vi "EKGTest.vi"() -> ()   [LabVIEW 2010]
uses:
  <instrlib>/niHWS/nihws.llb/niHWS Open File Permissions ID.ctl
  Fear Conditioning/GlobalFear.vi
  <instrlib>/niHWS/nihws.llb/niHWS Write Digital U32.vi
  <instrlib>/niHWS/nihws.llb/niHWS Write Analog DBL.vi
  <instrlib>/niHWS/nihws.llb/niHWS Write Analog WDT.vi
  <vilib>/measure/matone.llb/Extract Single Tone Information N Chan.vi
  <vilib>/measure/NI_MAPro.lvlib
panel:
  out "HR 3":dbl
  in  "Knob":dbl(knob) scale=7.0..15.0
  in  "stop":bool
  out "Filtered ECG Signal":waveform(dbl)[](graph)
  out "HR 2":dbl(graph)
  out "HR":dbl format="%#_4g"
  out "Detected HR":dynamicdata(graph)
  in  "HR % Change\nThreshold":dbl(slide)=25.0 scale=0.0..25.0
  out "Threshold":dbl
  out "Error Thr":dbl
  out "Skipped":bool
  in  "Rate Corrector":bool=TRUE
  in  "# average":dbl=20.0
  out "RAW ECG Signal":dynamicdata(graph)
  out "det Freq":dbl
  in  "Record":bool
  in  "Recording Path":path
  in  "Activity mouse":refnum<visa-resource-name>
  out "Activity monitor":dynamicdata(graph)
  in  "Mouse Axis":bool
  in  "DPI":dbl=350.0
  out "Cycles \ncompleted":dbl
  out "Shock":bool
  out "Audio":bool
  in  "Start":bool
  in  "stop 2":bool
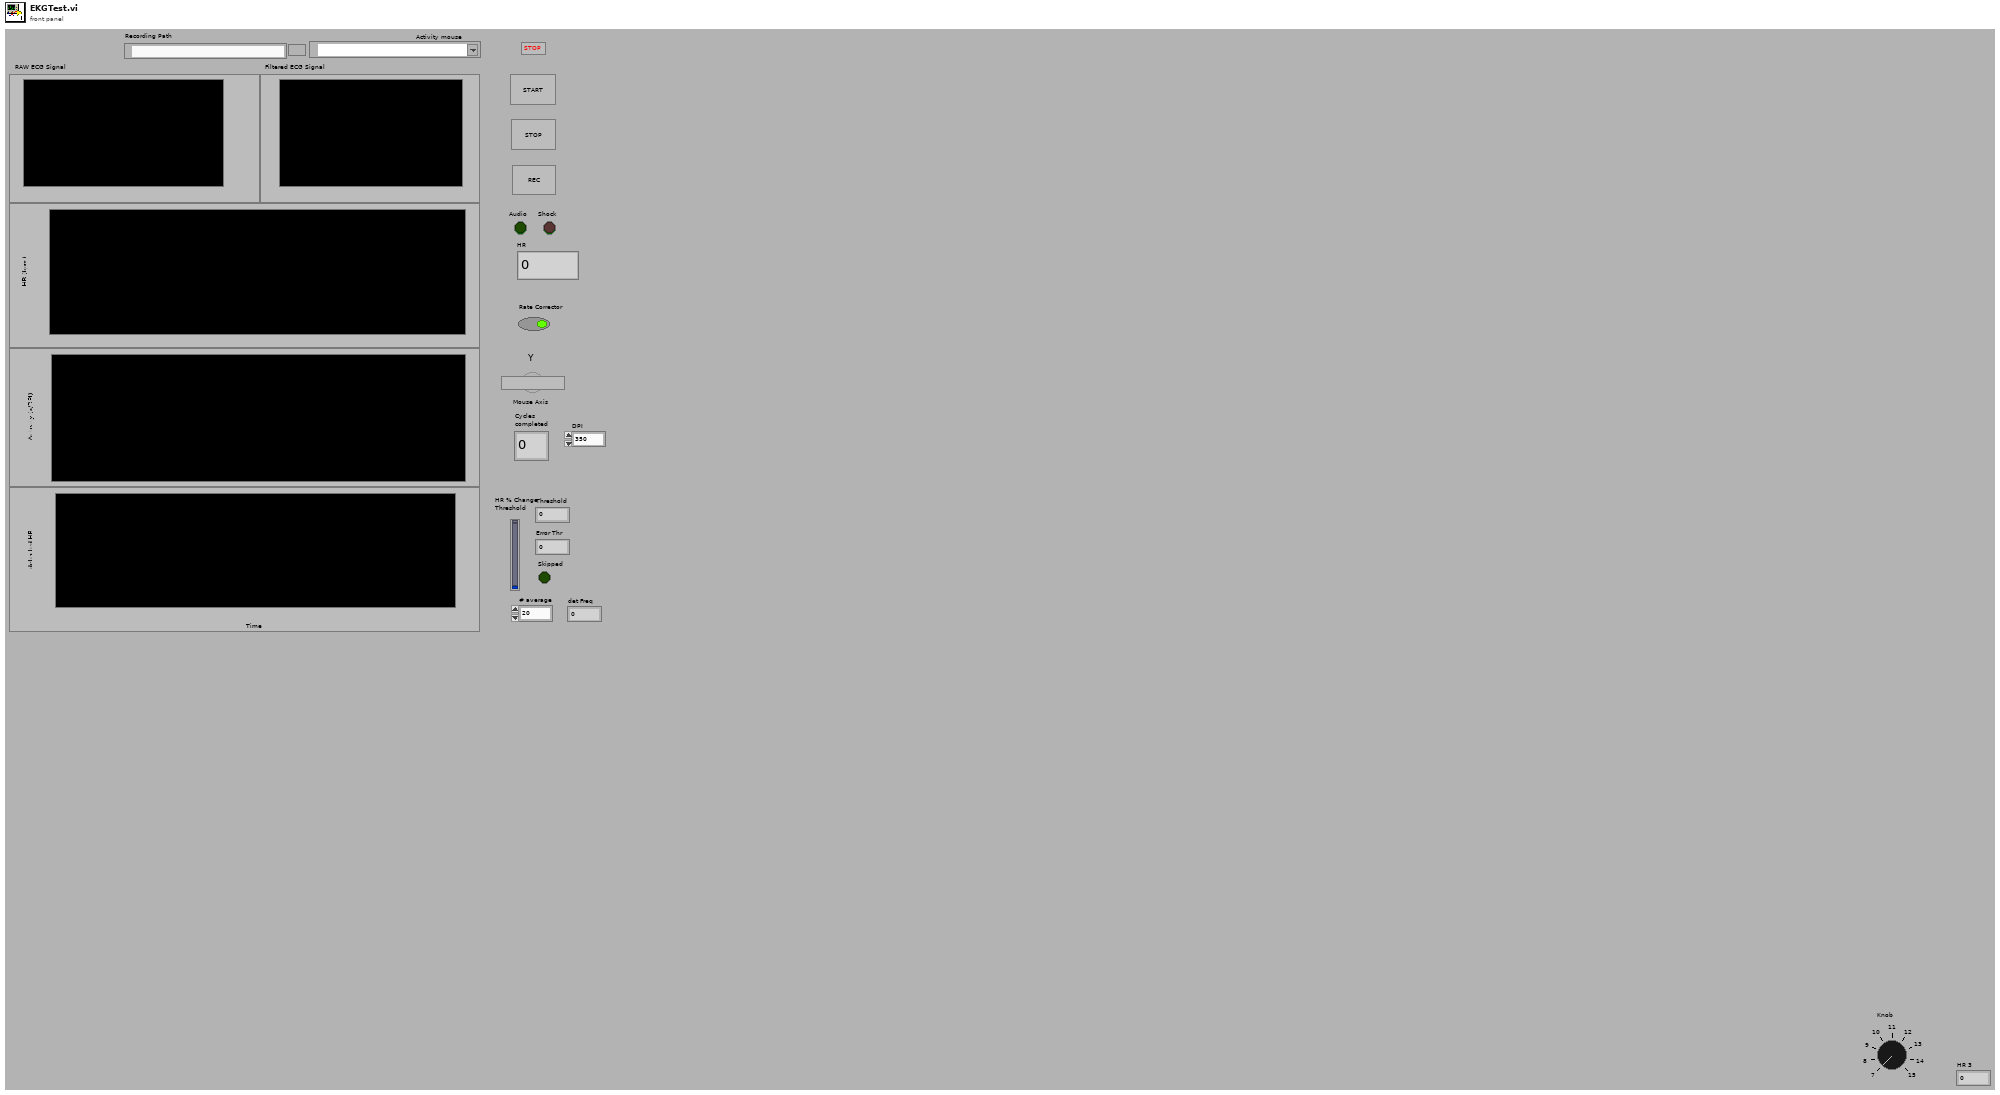
[diagram p1: front panel]
types:
  T1 = typedef "niHWS Open File Permissions ID.ctl" = enum32{"Read Only", "Read/Write Existing", "Read/Write/Create New", "Read/Write/Create New Always"}
  T2 = cluster{"approx freq. (optional)":dbl, "search (+/- % of Fsampl.)":dbl}
  T3 = cluster{"Array":dbl[], "Array 2":dbl[], "Array 3":dbl[], "Array 4":dbl[], "Array 5":dbl[], "Array 6":dbl[], "Array 7":dbl[], "Array 8":dbl[]}
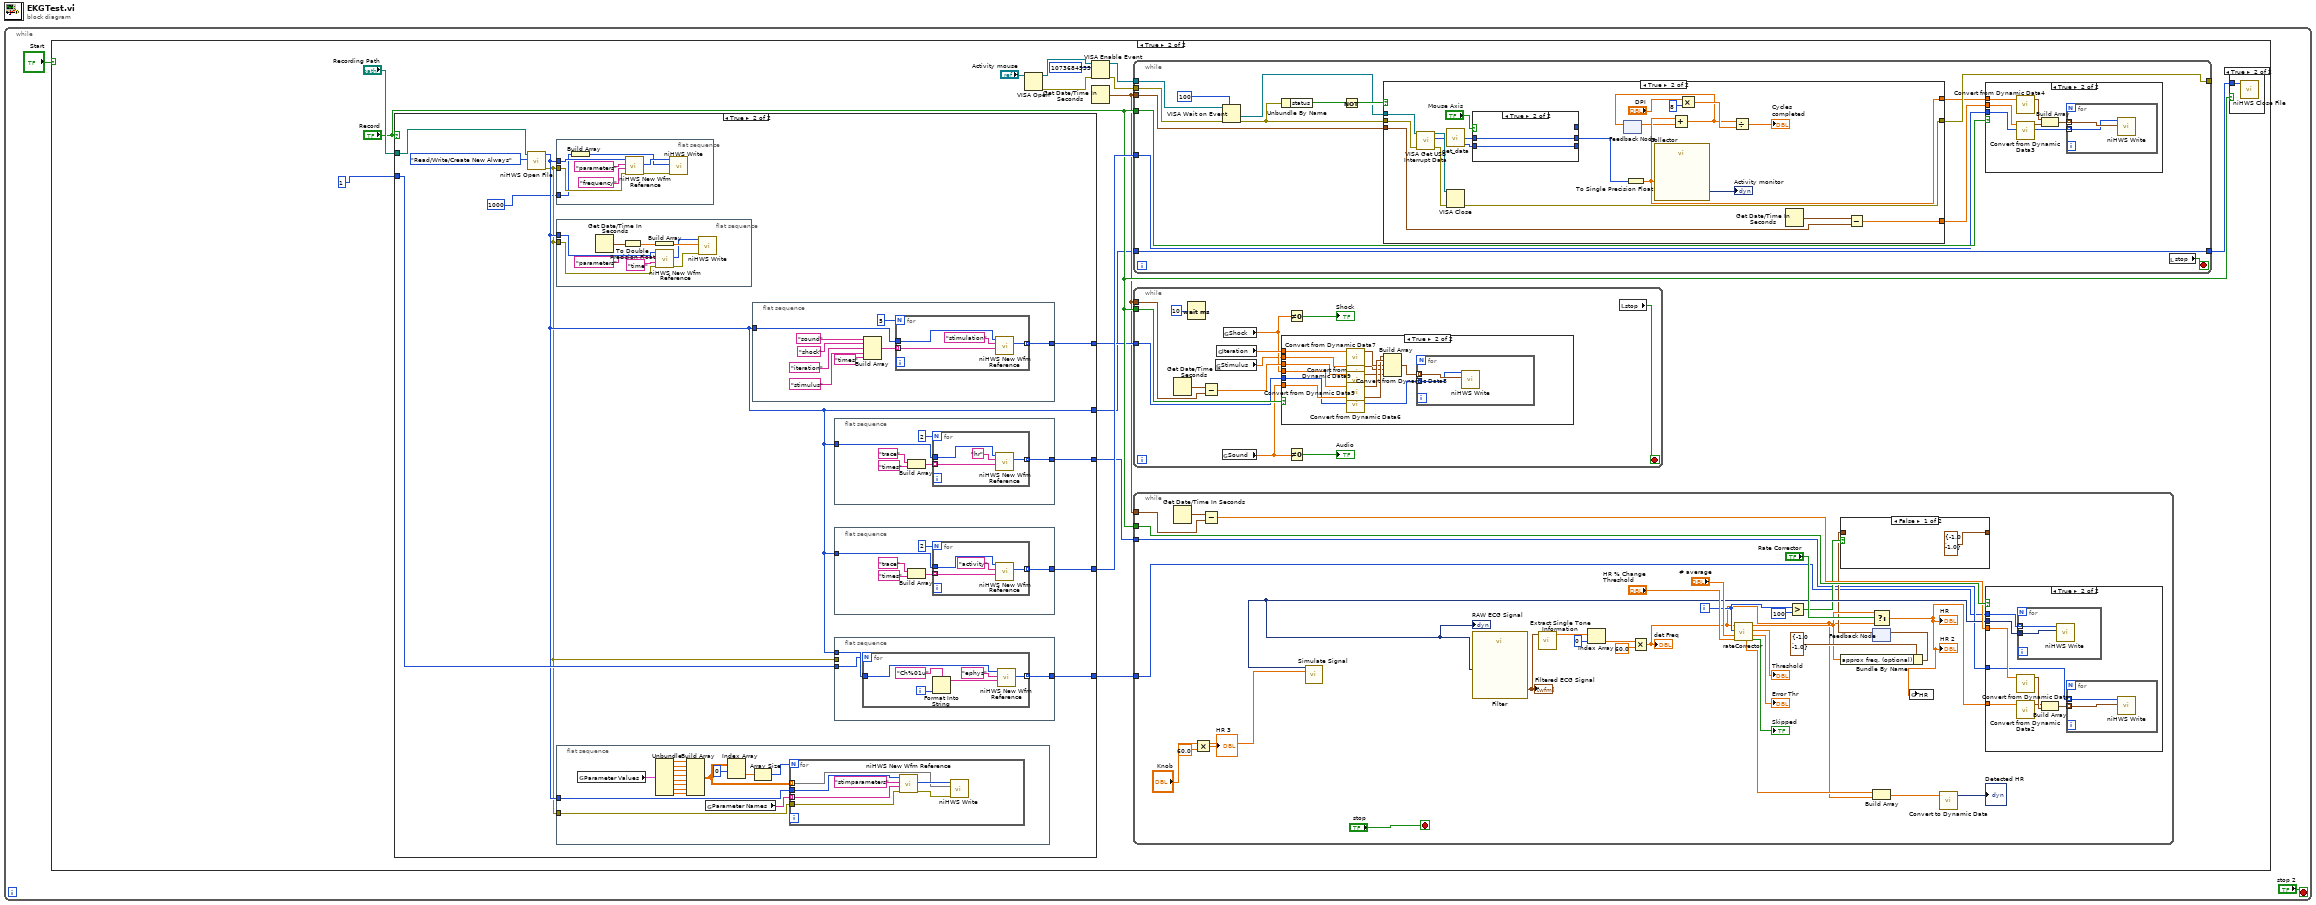
[diagram p0: block diagram]
diagram:
  n1 = while {
    stop <- "stop 2" stop-if-true
    n2 = case shown="True" "Start" {
      frame False {
      }
      frame True {
        n3 = case shown="True" "Record" {
          tunnel: 1 -> [_ w101]
          tunnel: "Recording Path" -> [_ w105]
          tunnel: [_ w103] -> w11
          tunnel: [_ w102] -> w9
          tunnel: [_ w99] -> w7
          tunnel: [_ w100] -> w5
          tunnel: [_ w97] -> w4
          frame False {
          }
          frame True {
            n4 = call <instrlib>:"niHWS Open File.vi"("permissions (0:read only)"=niHWS_Open_File_Permissions_ID."Read/Write/Create New Always", "file path"=w105) -> ("error out"=w98:errorcluster, "file handle"=w99:u32)  [unwired: 8 in]
            n5 = flat-sequence {
              tunnel: w98 -> [w160]
              tunnel: w99 -> [w159]
              tunnel: 1000 -> [w157]
              frame #0 {
                n6 = Build Array(w157) -> (w161:i32[])
                n7 = call <instrlib>:"niHWS New Wfm Reference.vi"("error in (no error)"=w160, "waveform name (empty)"="frequency" ("group name (empty)"), "group name (empty)"="parameters", "file handle in"=w159) -> ("error out"=w158:errorcluster, "waveform reference"=w164:u32)  [unwired: 5 in, 1 out]
                n8 = call-poly <instrlib>:"niHWS Write.vi"("error in (no error)"=w158, "data"=w161, "waveform reference in"=w164) -> ()  [unwired: 7 in, 2 out]
              }
            }
            n9 = flat-sequence {
              tunnel: w98 -> [w156]
              tunnel: w99 -> [w155]
              frame #0 {
                n10 = Get Date/Time In Seconds() -> (seconds since 1Jan1904=w154:timestamp)
                n11 = To Double Precision Float(number=w154) -> (double precision float=w153:dbl)
                n12 = Build Array(w153) -> (w152:dbl[])
                n13 = call <instrlib>:"niHWS New Wfm Reference.vi"("error in (no error)"=w156, "waveform name (empty)"="time" ("group name (empty)"), "group name (empty)"="parameters", "file handle in"=w155) -> ("error out"=w148:errorcluster, "waveform reference"=w149:u32)  [unwired: 5 in, 1 out]
                n14 = call-poly <instrlib>:"niHWS Write.vi"("error in (no error)"=w148, "data"=w152, "waveform reference in"=w149) -> ()  [unwired: 7 in, 2 out]
              }
            }
            n15 = flat-sequence {
              tunnel: w99 -> [w166]
              tunnel: w98 -> [w165]
              frame #0 {
                n16 = global read "GlobalFear.vi" "Parameter Values"() -> (w167:T3)
                n17 = Unbundle(w167) -> ("Array"=w168:dbl[], "Array 2"=w169:dbl[], "Array 3"=w170:dbl[], "Array 4"=w171:dbl[], "Array 5"=w172:dbl[], "Array 6"=w173:dbl[], "Array 7"=w174:dbl[], "Array 8"=w175:dbl[])
                n18 = Build Array(w168, w169, w170, w171, w172, w173, w174, w175) -> (w179:dbl[][])
                n19 = global read "GlobalFear.vi" "Parameter Names"() -> (w180:string[])
                n20 = Index Array(array=w179, index (row)=0) -> (element=w177:dbl[])  [unwired: 1 in]
                n21 = Array Size(array=w177) -> (size(s)=w176:i32)
                n22 = for {
                  N: w176 -> [_]
                  tunnel: w179 -> [w185] mode=indexing
                  tunnel: w180 -> [w184] mode=indexing
                  tunnel: w166 -> [w183]
                  tunnel: w165 -> [w182]
                  n23 = call <instrlib>:"niHWS New Wfm Reference.vi"("error in (no error)"=w182, "waveform name (empty)"=w184, "group name (empty)"="stimparameters", "file handle in"=w183) -> ("error out"=w181:errorcluster, "waveform reference"=w186:u32)  [unwired: 5 in, 1 out]
                  n24 = call-poly <instrlib>:"niHWS Write.vi"("error in (no error)"=w181, "data"=w185, "waveform reference in"=w186) -> ()  [unwired: 7 in, 2 out]
                }
              }
            }
            n25 = flat-sequence {
              tunnel: [w113] -> w102
              tunnel: w99 -> [w112]
              frame #0 {
                n26 = Build Array("sound" ("format string"), "shock" ("format string"), "iteration" ("format string"), "stimulus" ("format string"), "times") -> (w106:string[])
                n27 = for {
                  N: 5 -> [_]
                  tunnel: [w118] -> w113 mode=indexing
                  tunnel: w112 -> [w116]
                  tunnel: w106 -> [w115] mode=indexing
                  n28 = call <instrlib>:"niHWS New Wfm Reference.vi"("waveform name (empty)"=w115, "group name (empty)"="stimulation", "file handle in"=w116) -> ("waveform reference"=w118:u32)  [unwired: 6 in, 2 out]
                }
              }
            }
            n29 = flat-sequence {
              tunnel: [w123] -> w100
              tunnel: w99 -> [w122]
              frame #0 {
                n30 = Build Array("trace" ("format string"), "times" ("format string")) -> (w119:string[])
                n31 = for {
                  N: 2 -> [_]
                  tunnel: [w128] -> w123 mode=indexing
                  tunnel: w122 -> [w126]
                  tunnel: w119 -> [w125] mode=indexing
                  n32 = call <instrlib>:"niHWS New Wfm Reference.vi"("waveform name (empty)"=w125, "group name (empty)"="hr", "file handle in"=w126) -> ("waveform reference"=w128:u32)  [unwired: 6 in, 2 out]
                }
              }
            }
            n33 = flat-sequence {
              tunnel: [w134] -> w103
              tunnel: w99 -> [w133]
              frame #0 {
                n34 = Build Array("trace" ("format string"), "times" ("format string")) -> (w129:string[])
                n35 = for {
                  N: 2 -> [_]
                  tunnel: [w138] -> w134 mode=indexing
                  tunnel: w133 -> [w136]
                  tunnel: w129 -> [w135] mode=indexing
                  n36 = call <instrlib>:"niHWS New Wfm Reference.vi"("waveform name (empty)"=w135, "group name (empty)"="activity", "file handle in"=w136) -> ("waveform reference"=w138:u32)  [unwired: 6 in, 2 out]
                }
              }
            }
            n37 = flat-sequence {
              tunnel: w101 -> [w140]
              tunnel: w99 -> [w141]
              tunnel: w98 -> [_]
              tunnel: [w139] -> w97
              frame #0 {
                n38 = for {
                  N: w140 -> [_]
                  tunnel: [w142] -> w139 mode=indexing
                  tunnel: w141 -> [w147]
                  i -> [w145]
                  n39 = Format Into String(format string="Ch%01u", w145) -> (resulting string=w143:string)  [unwired: 2 in, 1 out]
                  n40 = call <instrlib>:"niHWS New Wfm Reference.vi"("waveform name (empty)"=w143, "group name (empty)"="ephys", "file handle in"=w147) -> ("waveform reference"=w142:u32)  [unwired: 6 in, 2 out]
                }
              }
            }
          }
        }
        n41 = VISA Open(VISA resource name="Activity mouse") -> (VISA resource name=w17:refnum<visa-resource-name>, error out=w16:errorcluster)  [unwired: 1 in, 3 out]
        n42 = VISA Enable Event(8:w16, 10:u32 1073684535 ("event type"), 11:w17) -> (0:w13:errorcluster, 3:w14:refnum<visa-resource-name>)  [unwired: 1 out]
        n43 = Get Date/Time In Seconds() -> (seconds since 1Jan1904=w8:timestamp)
        n44 = while {
          tunnel: w14 -> [w60]
          tunnel: w13 -> [w59]
          tunnel: w8 -> [w58]
          tunnel: [w52] -> _
          tunnel: "Record" -> [w51]
          tunnel: w11 -> [w48]
          tunnel: w7 -> [w46]
          tunnel: [w46] -> w6
          stop <- w47 stop-if-true
          n45 = VISA Wait on Event(7:u32 100 ("timeout (0)"), 8:w59, 11:w60) -> (0:w53:errorcluster, 1:w54:refnum<visa-resource-name>)  [unwired: 4 out]
          n46 = Unbundle By Name(w53) -> ("status"=w55:bool)
          n47 = Not(x=w55) -> (.not. x?=w56:bool)
          n48 = case shown="True" w56 {
            tunnel: w54 -> [_ w87]
            tunnel: [w69 w86] -> w52
            tunnel: w53 -> [w69 w85]
            tunnel: w58 -> [_ w83]
            tunnel: [_ w76] -> w50
            tunnel: [_ w82] -> w49
            frame False {
            }
            frame True {
              n49 = call <vilib>:"VISA Get USB Interrupt Data.vi"("error in (no error)"=w85, "VISA USB Intr Event"=w87) -> ("error out"=w88:errorcluster, "data buffer"=w84:u8[], "VISA USB Intr Event out"=w89:refnum<visa-resource-name>)  [unwired: 7 out]
              n50 = call "get_data.vi"("data buffer"=w84) -> ("X Value"=w79:i8, "Y Value"=w77:i8)  [unwired: 1 out]
              n51 = VISA Close(VISA resource name=w89, error in (no error)=w88) -> (error out=w86:errorcluster)
              n52 = case shown="True" "Mouse Axis" {
                tunnel: w79 -> [w91 w94]
                tunnel: [w92 w94] -> w78
                tunnel: w77 -> [w92 w93]
                tunnel: [w91 _] -> _
                tunnel: [_ w93] -> _
                frame False {
                }
                frame True {
                }
              }
              n53 = feedback #1() -> (w75:sgl)  [unwired: 1 in]
              n54 = To Single Precision Float(number=w78) -> (single precision float=w76:sgl)
              n55 = call "Collector"("Signals"=w76) -> ("Collected Signals"=→"Activity monitor":dynamicdata)  [unwired: 9 in, 1 out]
              n56 = Add(x=w76, y=w75) -> (x+y=w73:sgl)
              n57 = feedback-in #1(w73) -> ()
              n58 = Multiply(x="DPI", y=8) -> (x*y=w74:dbl)
              n59 = Divide(x=w73, y=w74) -> (x/y=→"Cycles \ncompleted":dbl)
              n60 = Get Date/Time In Seconds() -> (seconds since 1Jan1904=w90:timestamp)
              n61 = Subtract(x=w90, y=w83) -> (x-y=w82:dbl)
            }
          }
          n62 = case shown="True" w51 {
            tunnel: w50 -> [_ w63]
            tunnel: w49 -> [_ w62]
            tunnel: w48 -> [_ w61]
            frame False {
            }
            frame True {
              n63 = call "Convert from Dynamic Data4"("Dynamic Data Type"=w63) -> ("Waveform"=w64:waveform(dbl))  [unwired: 3 in]
              n64 = call "Convert from Dynamic Data3"("Dynamic Data Type"=w62) -> ("Waveform"=w65:waveform(dbl))  [unwired: 3 in]
              n65 = Build Array(w64, w65) -> (w66:waveform(dbl)[])
              n66 = for {
                tunnel: w66 -> [w68] mode=indexing
                tunnel: w61 -> [w67] mode=indexing
                n67 = call-poly <instrlib>:"niHWS Write.vi"("analog waveform"=w68, "waveform reference in"=w67) -> ()  [unwired: 8 in, 2 out]
              }
            }
          }
          n68 = local read "stop"() -> (w47:bool)
        }
        n69 = while {
          tunnel: "Record" -> [w30]
          tunnel: w9 -> [w29]
          tunnel: w8 -> [w27]
          stop <- w31 stop-if-true
          n70 = Get Date/Time In Seconds() -> (seconds since 1Jan1904=w28:timestamp)
          n71 = Wait (ms)(milliseconds to wait=10) -> ()  [unwired: 1 out]
          n72 = Subtract(x=w28, y=w27) -> (x-y=w26:dbl)
          n73 = global read "GlobalFear.vi" "Stimulus"() -> (w19:dbl)
          n74 = global read "GlobalFear.vi" "Iteration"() -> (w25:dbl)
          n75 = global read "GlobalFear.vi" "Sound"() -> (w24:dbl)
          n76 = global read "GlobalFear.vi" "Shock"() -> (w22:dbl)
          n77 = case shown="True" w30 {
            tunnel: w24 -> [_ w40]
            tunnel: w22 -> [_ w39]
            tunnel: w29 -> [_ w38]
            tunnel: w26 -> [_ w36]
            tunnel: w25 -> [_ w35]
            tunnel: w19 -> [_ w32]
            frame False {
            }
            frame True {
              n78 = call "Convert from Dynamic Data7"("Dynamic Data Type"=w35) -> ("Waveform"=w37:waveform(dbl))  [unwired: 3 in]
              n79 = call "Convert from Dynamic Data9"("Dynamic Data Type"=w32) -> ("Waveform"=w33:waveform(dbl))  [unwired: 3 in]
              n80 = call "Convert from Dynamic Data8"("Dynamic Data Type"=w36) -> ("Waveform"=w34:waveform(dbl))  [unwired: 3 in]
              n81 = call "Convert from Dynamic Data5"("Dynamic Data Type"=w39) -> ("Waveform"=w42:waveform(dbl))  [unwired: 3 in]
              n82 = call "Convert from Dynamic Data6"("Dynamic Data Type"=w40) -> ("Waveform"=w41:waveform(dbl))  [unwired: 3 in]
              n83 = Build Array(w41, w42, w37, w33, w34) -> (w43:waveform(dbl)[])
              n84 = for {
                tunnel: w43 -> [w45] mode=indexing
                tunnel: w38 -> [w44] mode=indexing
                n85 = call-poly <instrlib>:"niHWS Write.vi"("analog waveform"=w45, "waveform reference in"=w44) -> ()  [unwired: 8 in, 2 out]
              }
            }
          }
          n86 = Not Equal To 0?(x=w22) -> (x != 0?=→"Shock":bool)
          n87 = Not Equal To 0?(x=w24) -> (x != 0?=→"Audio":bool)
          n88 = local read "stop"() -> (w31:bool)
        }
        n89 = while {
          tunnel: "Record" -> [w221]
          tunnel: w8 -> [w215]
          tunnel: w5 -> [w194]
          tunnel: w4 -> [w193]
          i -> [w198]
          stop <- "stop" stop-if-true
          n90 = Get Date/Time In Seconds() -> (seconds since 1Jan1904=w216:timestamp)
          n91 = Multiply(x="Knob", y=60.0) -> (x*y=→"HR 3":dbl)
          n92 = Subtract(x=w216, y=w215) -> (x-y=w214:dbl)
          n93 = call "Simulate Signal"("Frequency"="Knob") -> ("Square with Gamma Noise"=w200:dynamicdata)  [unwired: 13 in, 1 out]
          "RAW ECG Signal" <- w200
          n94 = call "Filter"("input signals"=w200) -> ("filtered data"=w217:waveform(dbl)[])  [unwired: 17 in, 1 out]
          "Filtered ECG Signal" <- w217
          n95 = call-poly <vilib>:"Extract Single Tone Information.vi"("time signals in"=w217) -> ("detected frequencies"=w220:dbl[])  [unwired: 5 in, 5 out]
          n96 = Index Array(array=w220, index=0) -> (element=w203:dbl)
          n97 = Multiply(x=w203, y=60.0) -> (x*y=w195:dbl)
          "det Freq" <- w195
          n98 = call "rateCorrector.vi"("threshold"="HR % Change\nThreshold", "intergration"="# average", "count"=w198, "HR"=w195) -> ("skipped"=→"Skipped":bool, "error count"=→"Error Thr":dbl, "actual threshold"=→"Threshold":dbl, "HR"=w201:dbl, "Raw corr"=w205:dbl)  [unwired: 3 in]
          n99 = Greater?(x=w198, y=100 ("index")) -> (0:w197:bool)
          n100 = Bundle By Name(cluster=T2 {"approx freq. (optional)"=-1.0, "search (+/- % of Fsampl.)"=-1.0} ("advanced search"), "approx freq. (optional)"=w201) -> (w202:T2)
          n101 = Select(t=w201, s="Rate Corrector", f=w195) -> (s? t:f=w188:dbl)
          "HR 2" <- w188
          "HR" <- w188
          n102 = feedback-in #2(w202) -> ()
          n103 = feedback #2() -> (w196:T2)  [unwired: 1 in]
          n104 = case shown="False" w197 {
            tunnel: [T2 {"approx freq. (optional)"=-1.0, "search (+/- % of Fsampl.)"=-1.0} ("advanced search") w223] -> _
            tunnel: w196 -> [_ w223]
            frame False {
            }
            frame True {
            }
          }
          n105 = Build Array(w205, w195) -> (w207:dbl[])
          n106 = global write "GlobalFear.vi" "HR"(w188) -> ()
          n107 = call "Convert to Dynamic Data"("Array"=w207) -> ("Dynamic Data Type"=→"Detected HR":dynamicdata)  [unwired: 3 in]
          n108 = case shown="True" w221 {
            tunnel: w200 -> [_ w231]
            tunnel: w214 -> [_ w227]
            tunnel: w188 -> [_ w226]
            tunnel: w194 -> [_ w225]
            tunnel: w193 -> [_ w224]
            frame False {
            }
            frame True {
              n109 = call "Convert from Dynamic Data"("Dynamic Data Type"=w227) -> ("Waveform"=w230:waveform(dbl))  [unwired: 3 in]
              n110 = call "Convert from Dynamic Data2"("Dynamic Data Type"=w226) -> ("Waveform"=w229:waveform(dbl))  [unwired: 3 in]
              n111 = for {
                tunnel: w231 -> [w235]
                tunnel: w224 -> [w234] mode=indexing
                n112 = call-poly <instrlib>:"niHWS Write.vi"("analog waveform"=w235, "waveform reference in"=w234) -> ()  [unwired: 8 in, 2 out]
              }
              n113 = Build Array(w229, w230) -> (w228:waveform(dbl)[])
              n114 = for {
                tunnel: w228 -> [w233] mode=indexing
                tunnel: w225 -> [w232] mode=indexing
                n115 = call-poly <instrlib>:"niHWS Write.vi"("analog waveform"=w233, "waveform reference in"=w232) -> ()  [unwired: 8 in, 2 out]
              }
            }
          }
        }
        n116 = case shown="True" "Record" {
          tunnel: w6 -> [_ w95]
          frame False {
          }
          frame True {
            n117 = call <instrlib>:"niHWS Close File.vi"("file handle"=w95) -> ()  [unwired: 10 in, 1 out]
          }
        }
      }
    }
  }
